vi "Grid Measurements Example - ExtractPointSpectro.vi"(8 "error in (no error)":errorcluster, 9 "Channel index":i32, 10 "Experiment to read (Index)":i32, 11 "Binary Spectroscopy File":path) -> (0 "error out":errorcluster, 2 "Channel data":sgl[](array[numeric]) format="%#_6p", 3 "Spectro Points":dbl[](array[numeric]) format="%#_6p")   [LabVIEW 2017]
doc: "<B>Extracts a point spectroscopy curve (1 channel) from a binary spectroscopy file (.3ds).</B>\n\n<B>Binary Spectroscopy File</B>: path to 3ds file\n<B>Experiment to read (Index)</B>: index of point spectroscopy experiment. The index is 0-based.\n<B>Channel index</B>: index of the channel to extract.\n\n<B>Spectro Points</B>: values of sweep signal at which measurements were taken\n<B>Channel data</B>: values of the specified channel at the spectro points\n\n- Nanonis Programming Interface -"
uses:
  Nanonis Prog Interface.lvlib
panel:
  out "XY Graph":cluster{"Array":dbl[], "data":sgl[]}(graph)
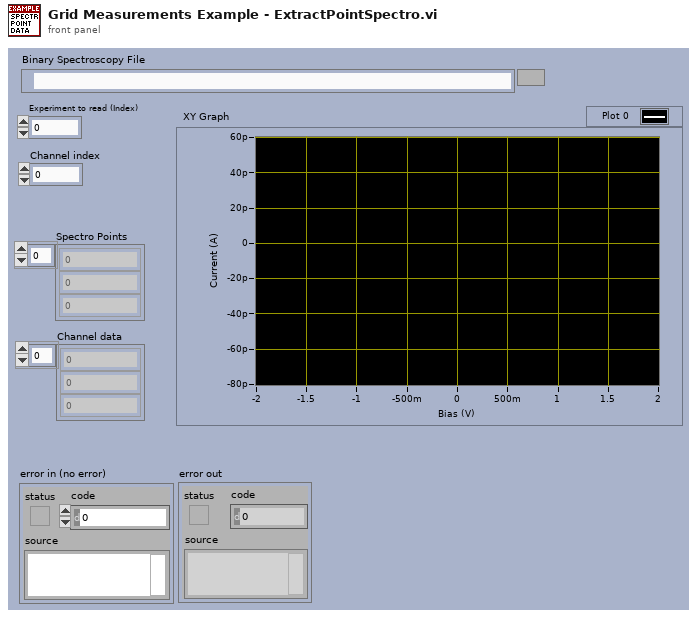
[diagram p1: front panel]
types:
  T1 = typedef "Nanonis Prog Interface.lvlib/Binary_SpectroscopyFile-Config.ctl" = cluster{"Num Par":i32, "Exp size":i32, "Points":i32, "Grid Dim X":i32, "Grid Dim Y":i32, "Header size":i32, "Channels":string[], "Parameters":string[], "Sweep Signal":string, "Grid":cluster{"center X (m)":sgl, "center Y (m)":sgl, "width (m)":sgl, "height (m)":sgl, "angle (deg)":sgl}}
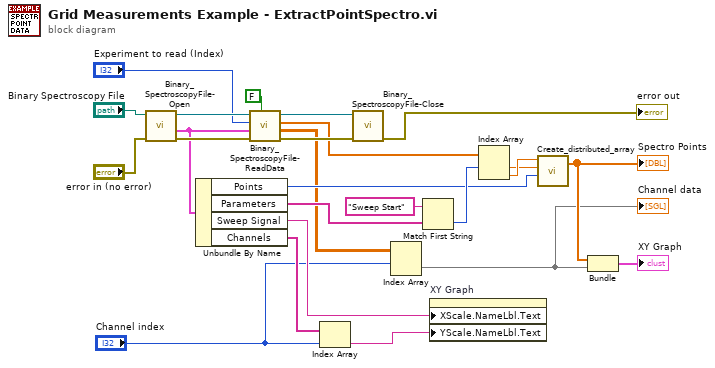
[diagram p0: block diagram]
diagram:
  n1 = call "Binary_SpectroscopyFile-Open.vi"("error in (no error)"="error in (no error)", "Binary Spectroscopy File"="Binary Spectroscopy File") -> ("error out"=w17:errorcluster, "Config"=w11:T1, "File ref"=w18:refnum<file>)  [unwired: 5 in, 2 out]
  n2 = Unbundle By Name(w11) -> ("Points"=w20:i32, "Parameters"=w21:string[], "Sweep Signal"=w6:string, "Channels"=w5:string[])
  n3 = call "Binary_SpectroscopyFile-ReadData.vi"("Read Parameters only? (F)"=FALSE, "error in"=w17, "Config"=w11, "Experiment to read (Index)"="Experiment to read (Index)", "File ref In"=w18) -> ("error out"=w14:errorcluster, "data"=w10:sgl[][], "Parameter values"=w13:sgl[], "File ref Out"=w15:refnum<file>)  [unwired: 3 in]
  n4 = Index Array(array=w5, index="Channel index") -> (element=w4:string)
  n5 = call "Binary_SpectroscopyFile-Close.vi"("error in"=w14, "File ref"=w15) -> ("error out"=→"error out":errorcluster)  [unwired: 9 in]
  n6 = Index Array(array=w10, index (row)="Channel index") -> (element=w8:sgl[])  [unwired: 1 in]
  "Channel data" <- w8
  n7 = Match First String(2:w21, 3:"Sweep Start" ("string")) -> (0:w24:i32)  [unwired: 1 out]
  n8 = property on="XY Graph" class="XYGraph (strict)"("XScale.NameLbl.Text"=w6, "YScale.NameLbl.Text"=w4) -> ()  [unwired: 2 in, 2 out]
  n9 = Index Array(array=w13, index #1=w24) -> (element #1=w22:sgl, element #2=w23:sgl)  [unwired: 1 in]
  n10 = call "Create_distributed_array.vi"("Upper Lim"=w23, "Lower Lim"=w22, "Num Points"=w20) -> ("Array"=w9:dbl[])  [unwired: 3 in]
  "Spectro Points" <- w9
  n11 = Bundle("Array"=w9, "data"=w8) -> (→"XY Graph":cluster{"Array":dbl[], "data":sgl[]})  [unwired: 1 in]
